vi "niRFUtil RFHS Channelizer CreateBuffer CSG.vi"(0 "Size":i32, 11 "error in (no error)":errorcluster) -> (4 "Buffer":csg[](array[numeric]), 6 "Embedded?":bool, 15 "error out":errorcluster)   [LabVIEW 2015, in "niRFUtil.lvlib"]
uses:
  niRFUtil.lvlib
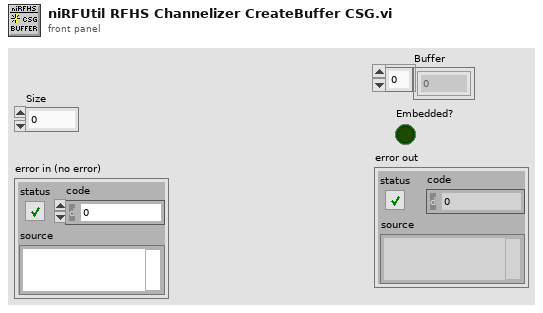
[diagram p1: front panel]
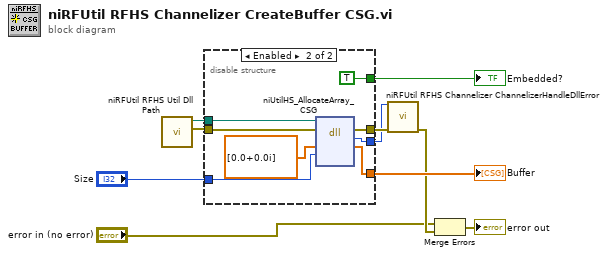
[diagram p0: block diagram]
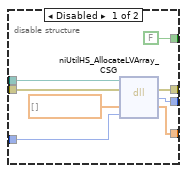
[diagram p2: hidden frame]
diagram:
  n1 = call "niRFUtil RFHS Util Dll Path.vi"() -> ("error out"=w4:errorcluster, "Path"=w10:path)  [unwired: 7 in, 3 out]
  n2 = disable-structure shown="Enabled" {
    disable-tunnel: w10 -> [w18 w25]
    disable-tunnel: "Size" -> [w17 w23]
    disable-tunnel: [w16 w24] -> w8
    disable-tunnel: w4 -> [w14 w22]
    disable-tunnel: [w13 w21] -> w6
    disable-tunnel: [FALSE ("Embedded?") TRUE] -> w7
    disable-tunnel: [w11 w19] -> w5
    frame Disabled {
      n3 = dll-call lib="?" fn="niUtilHS_AllocateLVArray_CSG"(path in=w18, error in=w14, "buf"=csg[] [] ("initialized array 6"), "length"=w17) -> (error out=w13:errorcluster, "return type"=w11:i32, "buf"=w16:csg[])  [unwired: 2 in, 1 out]
    }
    frame Enabled {
      n4 = dll-call lib="?" fn="niUtilHS_AllocateArray_CSG"(path in=w25, error in=w22, "buf"=csg[] [0.0+0.0i] ("initialized array 6"), "length"=w23) -> (error out=w21:errorcluster, "return type"=w19:i32, "buf"=w24:csg[])  [unwired: 4 in, 1 out]
    }
  }
  "Buffer" <- w8
  "Embedded?" <- w7
  n5 = call "niRFUtil RFHS Channelizer ChannelizerHandleDllError.vi"("Error"=w5, "error in (no error)"=w6) -> ("error out"=w2:errorcluster)  [unwired: 13 in]
  n6 = Merge Errors("error in (no error)", w2) -> (→"error out":errorcluster)
